vi "FRCts20_Backend_Shutdown.vi"(8 "error in (no error)":errorcluster, 11 "Engine_Refnums":T1) -> (0 "error out":errorcluster)   [LabVIEW 2013, in "FRCts20_Backend_Engine.lvlib"]
doc: "Releases all queues, closes db connection."
uses:
  FRCts20_Backend_Engine.lvlib
  FRCts20_Backend_EngineRefnums.ctl
  INI_Accessor/FRCts20_Backend_INI Controller.lvclass
  Dependencies/AMC/_SubVIs/TypeDefs/Message Queue.ctl
  Dependencies/AMC/_SubVIs/TypeDefs/Message.ctl
  Dependencies/Keyed Array/KeyedArray.ctl
  <vilib>/addons/database/Connection.llb/Conn ObjectReference.ctl
  FRCts20_Backend_Dyn_FGV_Command.ctl
  Dependencies/AMC/AMC.lvlib
  <vilib>/addons/database/NI_Database_API.lvlib
  Dependencies/Keyed Array/Tools_KeyedArray.lvlib
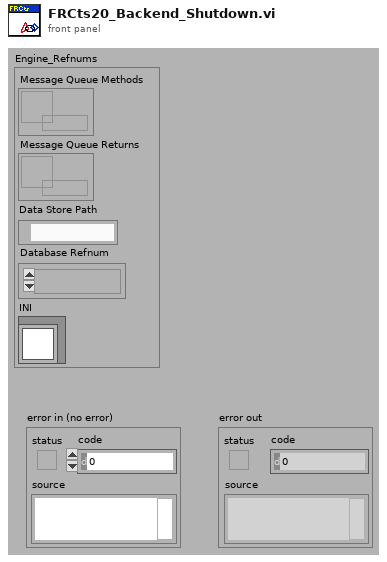
[diagram p1: front panel]
types:
  T1 = typedef "FRCts20_Backend_Engine.lvlib/FRCts20_Backend_EngineRefnums.ctl" = cluster{"Message Queue Methods":T2, "Message Queue Returns":T2, "Data Store Path":path, "Database Refnum":T3, "INI":refnum<class "FRCts20_Backend_INI Controller.lvclass">}
  T2 = typedef "AMC.lvlib/Message Queue.ctl" = refnum<queue>
  T3 = typedef "NI_Database_API.lvlib/Conn ObjectReference.ctl" = refnum<k1>
  T4 = typedef "FRCts20_Backend_Engine.lvlib/FRCts20_Backend_Dyn_FGV_Command.ctl" = enum16{"Load", "Locate", "Unload"}
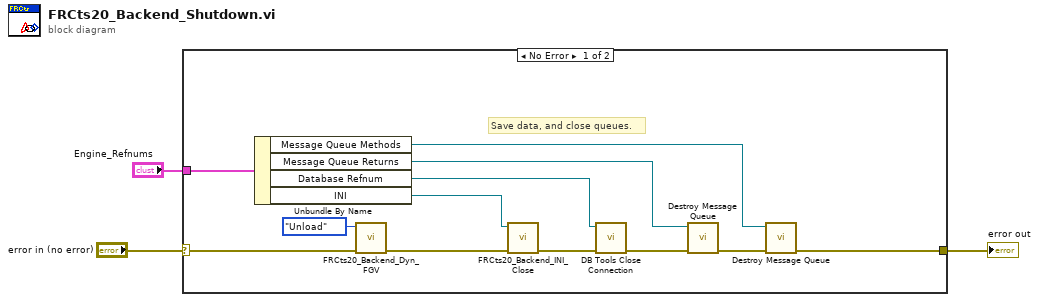
[diagram p0: block diagram]
diagram:
  n1 = case shown="No Error" "error in (no error)" {
    selector: "error in (no error)" -> [w8 w16]
    tunnel: [w11 w16] -> w2
    tunnel: "Engine_Refnums" -> [w15 _]
    frame No Error {
      # "Save data, and close queues."
      n2 = Unbundle By Name(w15) -> ("Message Queue Methods"=w12:T2, "Message Queue Returns"=w13:T2, "Database Refnum"=w9:T3, "INI"=w4:refnum<class "FRCts20_Backend_INI Controller.lvclass">)
      n3 = call "FRCts20_Backend_Dyn_FGV.vi"("error in"=w8, "Command"=FRCts20_Backend_Dyn_FGV_Command."Unload") -> ("error out"=w6:errorcluster)  [unwired: 7 in, 2 out]
      n4 = call "FRCts20_Backend_INI_Close.vi"("error in (no error)"=w6, "INI Controller in"=w4) -> ("error out"=w5:errorcluster)  [unwired: 7 in, 2 out]
      n5 = call <vilib>:"DB Tools Close Connection.vi"("error in (no error)"=w5, "connection reference"=w9) -> ("error out"=w10:errorcluster)  [unwired: 5 in]
      n6 = call "Destroy Message Queue.vi"("error in (no error)"=w10, "Message Queue in"=w13) -> ("error out"=w14:errorcluster)  [unwired: 8 in, 1 out]
      n7 = call "Destroy Message Queue.vi"("error in (no error)"=w14, "Message Queue in"=w12) -> ("error out"=w11:errorcluster)  [unwired: 8 in, 1 out]
    }
    frame Error {
    }
  }
  "error out" <- w2
